vi "S2DS_ClearBuffer.vi"(3 "Buffer length in":i32, 4 "Data array in":dbl[][](array[numeric]), 5 "Clear Buffer?":bool) -> (0 "Buffer length out":i32, 1 "Data array out":dbl[][](array[numeric]))   [LabVIEW 2025]
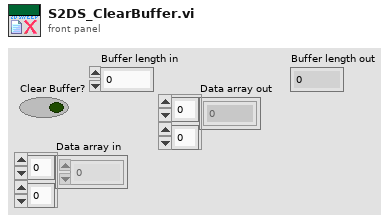
[diagram p1: front panel]
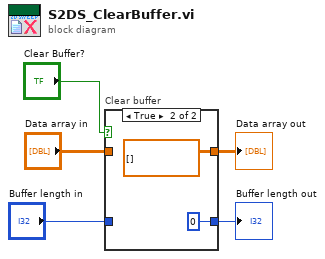
[diagram p0: block diagram]
diagram:
  n1 = case "Clear buffer" shown="True" "Clear Buffer?" {
    tunnel: [w7 dbl[][] []] -> w4
    tunnel: "Data array in" -> [w7 _]
    tunnel: [w6 0 ("Buffer length in")] -> w1
    tunnel: "Buffer length in" -> [w6 _]
    frame False {
    }
    frame True {
    }
  }
  "Data array out" <- w4
  "Buffer length out" <- w1
